vi "Apply Tombstone.vi"(8 "Error In":errorcluster) -> (0 "Error Out":errorcluster)   [LabVIEW 2017, in "Tests.lvlib" / "Toolkit.lvlib"]
uses:
  Toolkit.lvlib
  <vilib>/Utility/traverseref.llb/TRef TravTarget.ctl
  src/Toolkit/Typedefs/Bookmark Tags.ctl
  <vilib>/addons/_JKI Toolkits/Caraya/classes/Test/Test.lvclass
  <vilib>/Utility/traverseref.llb/VI Scripting - Traverse.lvlib
  <vilib>/addons/_JKI Toolkits/Caraya/classes/Assert/Assert.lvclass
  src/Toolkit/Toolkit.lvlib
  Tests.lvlib
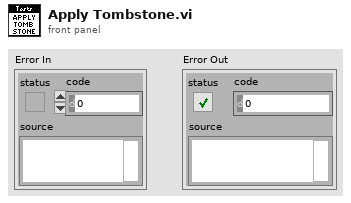
[diagram p1: front panel]
types:
  T1 = typedef "Toolkit.lvlib/Bookmark Tags.ctl" = enum16{"RIP", "Zombie"}
  T2 = typedef "TRef TravTarget.ctl" = enum16{"FP", "BD", "Other"}
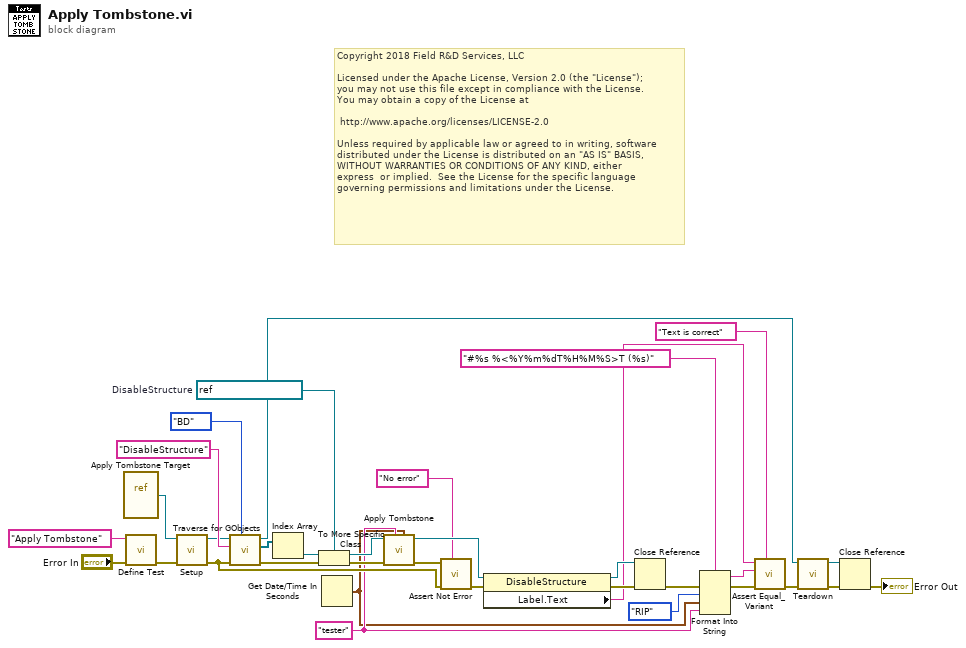
[diagram p0: block diagram]
diagram:
  w5 = "tester" ("Grave Digger")
  w28 = refnum<vi> refnum  # DisableStructure
  # "Copyright 2018 Field R&D Services, LLC\n\nLicensed under the Apache License, Version 2.0 (the \"License\");\nyou may not use this file except in compliance with the License.\nYou may obtain a copy of the License at\n\n\thttp://www.apache.org/licenses/LICENSE-2.0\n\nUnless required by applicable law or agreed to in writing, software\ndistributed under the License is distributed on an \"AS IS\" BASIS,\nWITHOUT WARRANTIES OR CONDITIONS OF ANY KIND, either \nexpress  or implied.  See the License for the specific language \ngoverning permissions and limitations under the License."
  n1 = vi-ref "Apply Tombstone Target.vi"() -> (w26:refnum<vi>)
  n2 = call <vilib>:"Define Test.vi"("error in (no error)"="Error In", "Label (VI Title)"="Apply Tombstone") -> ("error out"=w18:errorcluster)  [unwired: 9 in]
  n3 = call "Setup.vi"("Error In"=w18, "VI In"=w26) -> ("Error Out"=w13:errorcluster, "VI Out"=w25:refnum<vi>)  [unwired: 8 in]
  n4 = call <vilib>:"Traverse for GObjects.vi"("Traverse Target"=TRef_TravTarget."BD", "error in (no error)"=w13, "Class Name"="DisableStructure", "VI Refnum"=w25) -> ("error out"=w31:errorcluster, "References"=w30:refnum<vi>[], "dup VI Refnum"=w24:refnum<vi>)  [unwired: 4 in, 1 out]
  n5 = Index Array(array=w30) -> (element=w29:refnum<vi>)  [unwired: 1 in]
  n6 = To More Specific Class(target class=w28, reference=w29, error in=w31) -> (specific class reference=w27:refnum<vi>, error out=w14:errorcluster)
  n7 = Get Date/Time In Seconds() -> (seconds since 1Jan1904=w1:timestamp)
  n8 = call "Apply Tombstone.vi"("Time of Death (ToD)"=w1, "Grave Digger"=w5, "Error In"=w14, "Grave In"=w27) -> ("Error Out"=w11:errorcluster, "Grave Out"=w20:refnum<vi>)  [unwired: 6 in]
  n9 = call <vilib>:"Assert Not Error.vi"("Label"="No error", "error in (no error)"=w13, "Not Error?"=w11) -> ("error out"=w12:errorcluster)  [unwired: 8 in]
  n10 = property class="DisableStructure"(reference=w20, error in=w12) -> (reference out=w19:refnum<vi>, error out=w17:errorcluster, "Label.Text"=w2:string)
  n11 = Close Reference(reference=w19, error in (no error)=w17) -> (error out=w8:errorcluster)
  n12 = Format Into String(format string="#%s %<%Y%m%dT%H%M%S>T (%s)", error in=w8, Bookmark_Tags."RIP" ("Bookmark Tag"), w1, w5) -> (resulting string=w3:string, error out=w7:errorcluster)  [unwired: 1 in]
  n13 = call <vilib>:"Assert Equal_Variant.vi"("Label"="Text is correct", "error in (no error)"=w7, "Y"=w3, "X"=w2) -> ("error out"=w15:errorcluster)  [unwired: 7 in]
  n14 = call "Teardown.vi"("Error In"=w15, "VI In"=w24) -> ("Error Out"=w22:errorcluster, "VI Out"=w23:refnum<vi>)  [unwired: 8 in]
  n15 = Close Reference(reference=w23, error in (no error)=w22) -> (error out=→"Error Out":errorcluster)
